vi "niRFSTS SG Set Waveform Data.vi"(0 "TSM Context in":T1, 1 "Waveform Name":string, 7 "Waveform":cluster{"x0":dbl, "dx":dbl, "y":csg[]} {"y" format="%.2f"; "dx" format="%^.2e"; "x0" format="%^.2e"}, 11 "error in (no error)":errorcluster) -> (4 "TSM Context out":T1, 15 "error out":errorcluster)   [LabVIEW 2014]
uses:
  <vilib>/NI_TestStand_SemiconductorModule/NI_TestStand_Semiconductor_Module.lvlibp/PinMap/General/SemiconductorModuleContext.ctl
  <vilib>/NI_TestStand_SemiconductorModule/NI_TestStand_Semiconductor_Module.lvlibp
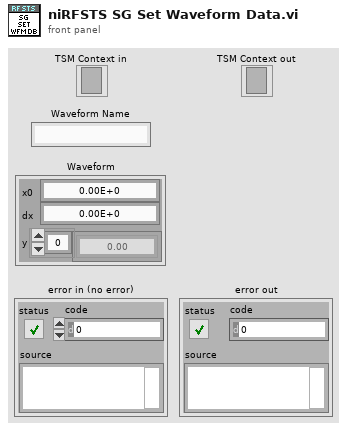
[diagram p1: front panel]
types:
  T1 = typedef "NI_TestStand_Semiconductor_Module.lvlibp/SemiconductorModuleContext.ctl" = refnum<k7>
  T2 = cluster{"Waveform DVR":refnum<data-value>, "Waveform Max Amplitude (V)":sgl}
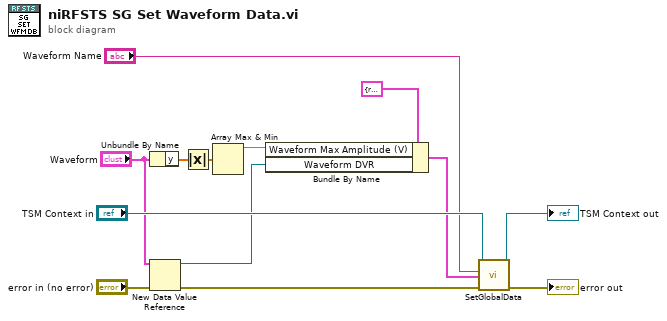
[diagram p0: block diagram]
diagram:
  n1 = Unbundle By Name("Waveform") -> ("y"=w9:csg[])
  n2 = New Data Value Reference(data value="Waveform", error in="error in (no error)") -> (data value reference=w4:refnum<data-value>)  [unwired: 1 out]
  n3 = Absolute Value(x=w9) -> (abs(x)=w8:sgl[])
  n4 = Array Max & Min(array=w8) -> (max value=w7:sgl)  [unwired: 3 out]
  n5 = Bundle By Name(cluster=T2 {"Waveform DVR"=refnum, "Waveform Max Amplitude (V)"=-1.0} ("SG Waveform DB Entry"), "Waveform Max Amplitude (V)"=w7, "Waveform DVR"=w4) -> (w3:T2)
  n6 = call <vilib>:"SetGlobalData.vi"("error in (no error)"="error in (no error)", "Data"=w3, "Data Id"="Waveform Name", "Semiconductor Module Context"="TSM Context in") -> ("error out"=→"error out":errorcluster, "Semiconductor Module Context Out"=→"TSM Context out":T1)  [unwired: 5 in]
